vi "Untitled 2.vi"() -> ()   [LabVIEW 2020]
uses:
  <vilib>/Instr/_visa.llb/VISA Configure Serial Port (Instr).vi
panel:
  in  "stop":bool
  in  "WriteBuffer":string
  out "concatenated string 2":string
  out "concatenated string":string
  in  "Boolean 2":bool
  in  "Boolean":bool
  in  "VISA resource name":refnum<visa-resource-name>
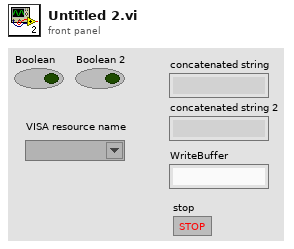
[diagram p1: front panel]
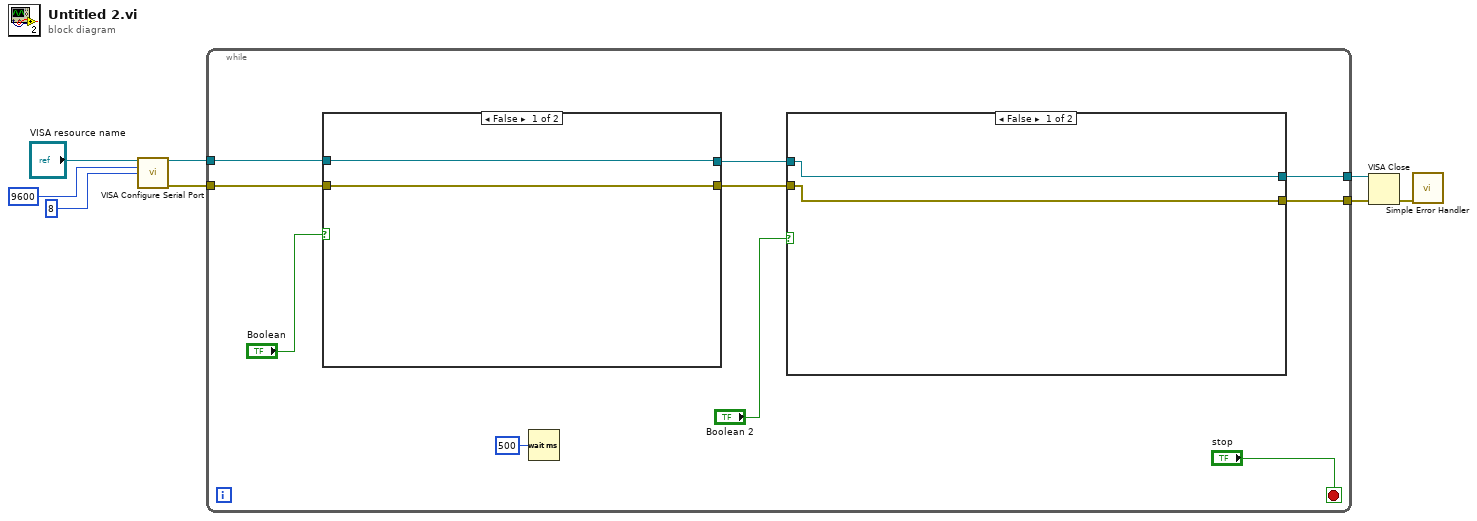
[diagram p0: block diagram]
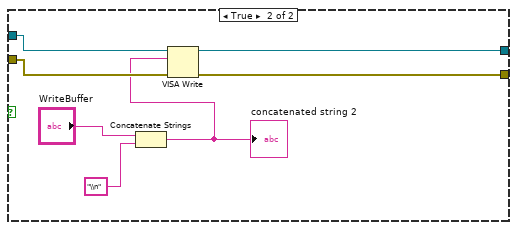
[diagram p2: hidden frame]
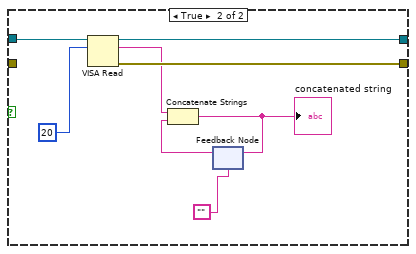
[diagram p3: hidden frame]
diagram:
  n1 = call-poly "VISA Configure Serial Port"("VISA resource name"="VISA resource name", "baud rate (9600)"=u32 9600, "data bits (8)"=u16 8) -> ("VISA resource name out"=w4:refnum<visa-resource-name>, "error out"=w5:errorcluster)  [unwired: 11 in]
  n2 = while {
    tunnel: w5 -> [w17]
    tunnel: w4 -> [w16]
    tunnel: [w12] -> w2
    tunnel: [w11] -> w3
    stop <- "stop" stop-if-true
    n3 = case shown="False" "Boolean" {
      tunnel: w17 -> [w28 _]
      tunnel: w16 -> [w29 w37]
      tunnel: [w29 w36] -> w14
      tunnel: [w28 w35] -> w13
      frame False {
      }
      frame True {
        n4 = VISA Read(VISA resource name=w37, byte count=u32 20) -> (VISA resource name out=w36:refnum<visa-resource-name>, read buffer=w33:string, error out=w35:errorcluster)  [unwired: 1 in, 1 out]
        n5 = feedback #1("") -> (w31:string)
        n6 = Concatenate Strings(w33, w31) -> (w32:string)
        "concatenated string" <- w32
        n7 = feedback-in #1(w32) -> ()
      }
    }
    n8 = Wait (ms)(milliseconds to wait=u32 500) -> ()  [unwired: 1 out]
    n9 = case shown="False" "Boolean 2" {
      tunnel: w14 -> [w20 w27]
      tunnel: w13 -> [w19 w26]
      tunnel: [w20 w25] -> w12
      tunnel: [w19 w24] -> w11
      frame False {
      }
      frame True {
        n10 = Concatenate Strings("WriteBuffer", "\\n" ("string")) -> (w23:string)
        "concatenated string 2" <- w23
        n11 = VISA Write(VISA resource name=w27, write buffer=w23, error in (no error)=w26) -> (VISA resource name out=w25:refnum<visa-resource-name>, error out=w24:errorcluster)  [unwired: 1 out]
      }
    }
  }
  n12 = VISA Close(VISA resource name=w2, error in (no error)=w3) -> (error out=w1:errorcluster)
  n13 = call <vilib>:"Simple Error Handler.vi"("error in (no error)"=w1) -> ()  [unwired: 4 in, 5 out]
